vi "Contour Line_Find Connected Contour Points Search.vi"(7 "Stack In":bool[](array[boolean]), 9 "index":i32, 10 "Intersected Edges":T2(array[cluster]), 11 "Contour Points":cluster{"x":dbl, "y":dbl}[](array[cluster])) -> (3 "Contour Segment":T1, 5 "Stack Out":bool[](array[boolean]))   [LabVIEW 2020, in "NI_AAL_Geometry.lvlib"]
uses:
  <vilib>/Analysis/NI_AAL_Geometry.lvlib
  <vilib>/Analysis/geometry.llb/Contour Line Segment.ctl
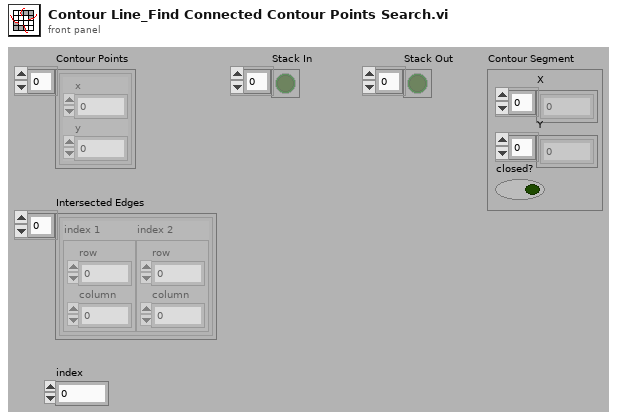
[diagram p1: front panel]
types:
  T1 = typedef "NI_AAL_Geometry.lvlib/Contour Line Segment.ctl" = cluster{"X":dbl[], "Y":dbl[], "closed?":bool}
  T2 = cluster{"index 1":cluster{"row":i32, "column":i32}, "index 2":cluster{"row":i32, "column":i32}}[]
  T3 = cluster{"index 1":cluster{"row":i32, "column":i32}, "index 2":cluster{"row":i32, "column":i32}}
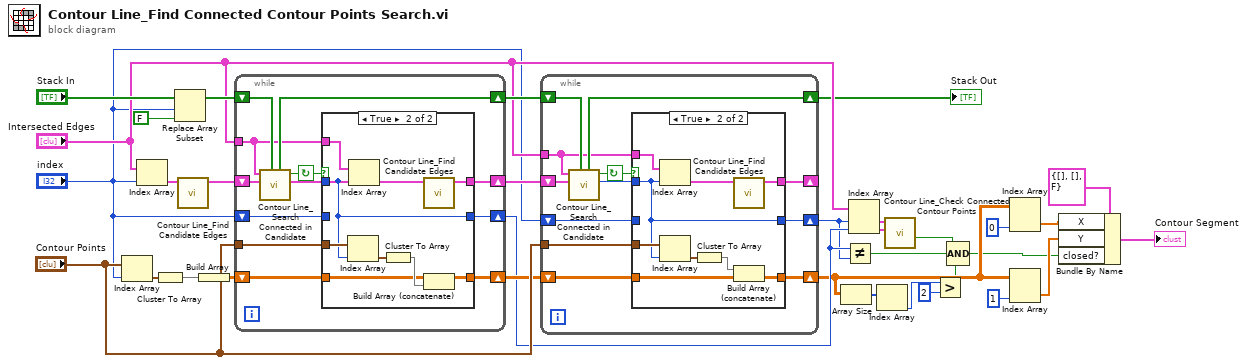
[diagram p0: block diagram]
diagram:
  n1 = Index Array(array="Contour Points", index="index") -> (element=w25:cluster{"x":dbl, "y":dbl})
  n2 = Index Array(array="Intersected Edges", index="index") -> (element=w29:T3)
  n3 = Cluster To Array(cluster=w25) -> (array=w26:dbl[])
  n4 = Replace Array Subset(array="Stack In", new element=FALSE ("new element/subarray"), index="index") -> (w23:bool[])
  n5 = call <vilib>:"Contour Line_Find Candidate Edges.vi"("edge"=w29) -> ("Candidate Edges"=w20:T2)  [unwired: 10 out]
  n6 = Build Array(w26) -> (w24:dbl[][])
  n7 = while {
    tunnel: "Intersected Edges" -> [w37]
    shift-right: [w40] -> w22
    shift-left: w23 -> [w41]
    tunnel: "Contour Points" -> [w44]
    shift-right: [w42] -> w18
    shift-left: w24 -> [w43]
    shift-right: [w35] -> _
    shift-left: w20 -> [w36]
    shift-right: [w33] -> w16
    shift-left: "index" -> [w34]
    stop <- w39 continue-if-true
    n8 = call <vilib>:"Contour Line_Search Connected in Candidate.vi"("Stack In"=w41, "Candidate Edges"=w36, "Intersected Edges"=w37) -> ("connected index"=w38:i32, "find?"=w39:bool, "Stack Out"=w40:bool[])  [unwired: 6 out]
    n9 = case shown="True" w39 {
      tunnel: w37 -> [_ w50]
      tunnel: w38 -> [_ w47]
      tunnel: w44 -> [_ w53]
      tunnel: w43 -> [w46 w52]
      tunnel: [w46 w51] -> w42
      tunnel: [_ w48] -> w35
      tunnel: w34 -> [w45 _]
      tunnel: [w45 w47] -> w33
      frame False {
      }
      frame True {
        n10 = Index Array(array=w53, index=w47) -> (element=w54:cluster{"x":dbl, "y":dbl})
        n11 = Index Array(array=w50, index=w47) -> (element=w49:T3)
        n12 = Cluster To Array(cluster=w54) -> (array=w55:dbl[])
        n13 = call <vilib>:"Contour Line_Find Candidate Edges.vi"("edge"=w49) -> ("Candidate Edges"=w48:T2)  [unwired: 10 out]
        n14 = Build Array (concatenate)(w52, w55) -> (w51:dbl[][])
      }
    }
  }
  n15 = while {
    tunnel: "Intersected Edges" -> [w60]
    shift-right: [w63] -> w13
    shift-left: w22 -> [w64]
    tunnel: "Contour Points" -> [w67]
    shift-right: [w65] -> w14
    shift-left: w18 -> [w66]
    shift-right: [w58] -> _
    shift-left: w20 -> [w59]
    shift-right: [w56] -> w15
    shift-left: "index" -> [w57]
    stop <- w62 continue-if-true
    n16 = call <vilib>:"Contour Line_Search Connected in Candidate.vi"("Stack In"=w64, "Candidate Edges"=w59, "Intersected Edges"=w60) -> ("connected index"=w61:i32, "find?"=w62:bool, "Stack Out"=w63:bool[])  [unwired: 6 out]
    n17 = case shown="True" w62 {
      tunnel: w60 -> [_ w73]
      tunnel: w61 -> [_ w70]
      tunnel: w67 -> [_ w76]
      tunnel: w66 -> [w69 w75]
      tunnel: [w69 w74] -> w65
      tunnel: [_ w71] -> w58
      tunnel: w57 -> [w68 _]
      tunnel: [w68 w70] -> w56
      frame False {
      }
      frame True {
        n18 = Index Array(array=w73, index=w70) -> (element=w72:T3)
        n19 = Index Array(array=w76, index=w70) -> (element=w77:cluster{"x":dbl, "y":dbl})
        n20 = Cluster To Array(cluster=w77) -> (array=w78:dbl[])
        n21 = call <vilib>:"Contour Line_Find Candidate Edges.vi"("edge"=w72) -> ("Candidate Edges"=w71:T2)  [unwired: 10 out]
        n22 = Build Array (concatenate)(w78, w75) -> (w74:dbl[][])
      }
    }
  }
  "Stack Out" <- w13
  n23 = Array Size(array=w14) -> (size(s)=w32:i32[])
  n24 = Not Equal?(x=w16, y=w15) -> (x != y?=w7:bool)
  n25 = Index Array(array="Intersected Edges", index #1=w15, index #2=w16) -> (element #1=w31:T3, element #2=w30:T3)
  n26 = Index Array(array=w32) -> (element=w10:i32)  [unwired: 1 in]
  n27 = call <vilib>:"Contour Line_Check Connected Contour Points.vi"("edge 2"=w30, "edge 1"=w31) -> ("connected?"=w8:bool)  [unwired: 9 out]
  n28 = Greater?(x=w10, y=2) -> (0:w6:bool)
  n29 = Compound Arithmetic op=AND(w8, w7, w6) -> (w1:bool)
  n30 = Index Array(array=w14, index (col)=0 ("disabled index (col)")) -> (element=w3:dbl[])  [unwired: 1 in]
  n31 = Index Array(array=w14, index (col)=1 ("disabled index (col)")) -> (element=w2:dbl[])  [unwired: 1 in]
  n32 = Bundle By Name(cluster=T1 {"X"=[], "Y"=[], "closed?"=FALSE} ("Contour Segment"), "X"=w3, "Y"=w2, "closed?"=w1) -> (→"Contour Segment":T1)
